vi "WLAN_be_EVM_SA_RS_CMP200.vi"(6 "SG Power":i32=-10, 7 "Function":T1, 8 "error in":errorcluster, 11 "VISA IN":refnum<visa-resource-name>="TCPIP::Vince_Wu-NB::inst0::INSTR") -> (0 "error out":errorcluster, 1 "EVM":dbl format="%#.3g", 2 "Power":dbl format="%#.3g", 3 "IDN":string)   [LabVIEW 2023, in "R_S.lvlib"]
uses:
  R_S.lvlib
  CTL/LitePoint_EVM_SA.ctl
panel:
  out "Response":string
  out "String":string
  out "EVM_ALL_Carrier_Mean":string
  out "PPDU_Power_Mean":string
  out "VSA?":string
  # "TCPIP::Vince_Wu-NB::inst0::INSTR"
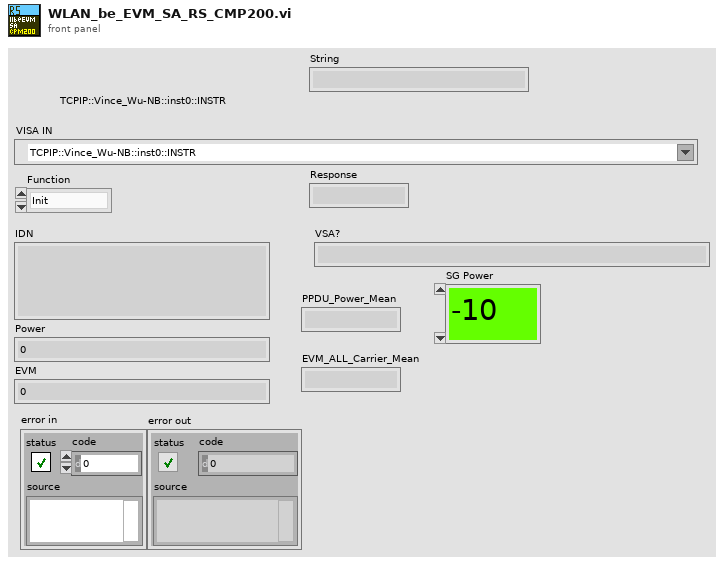
[diagram p1: front panel]
types:
  T1 = typedef "LitePoint_EVM_SA.ctl" = enum16{"Init", "Close", "set_SA", "get_EVM", "byPass", "getPower"}
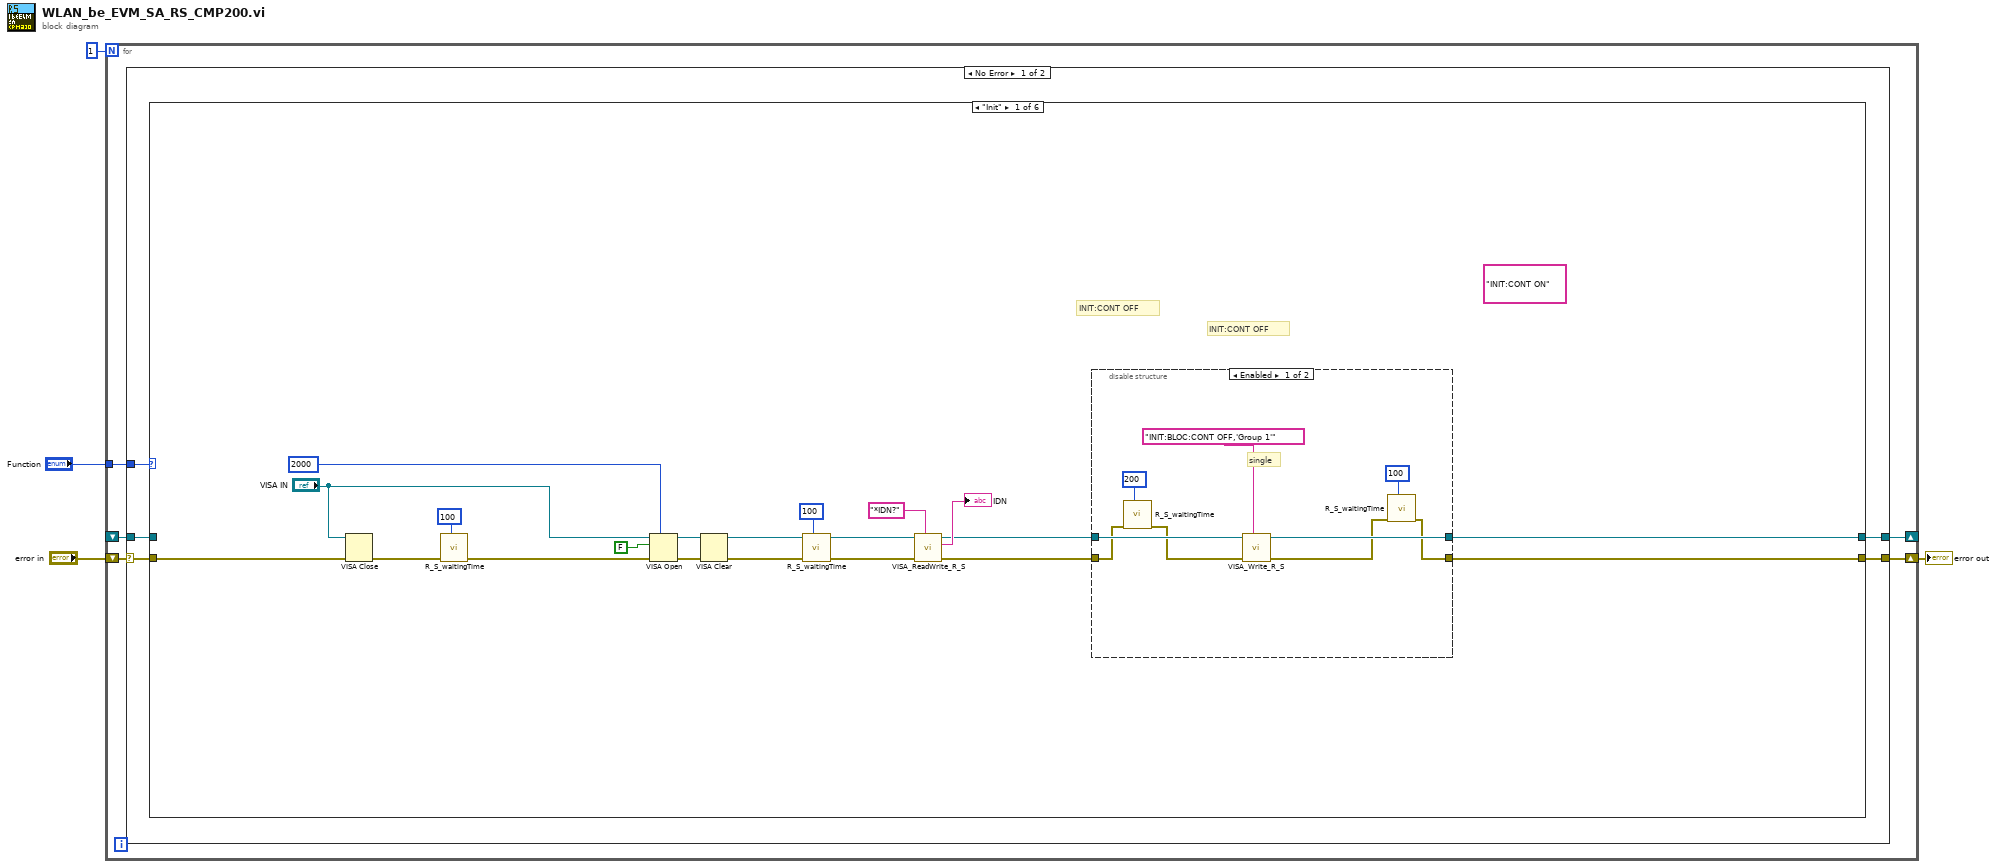
[diagram p0: block diagram]
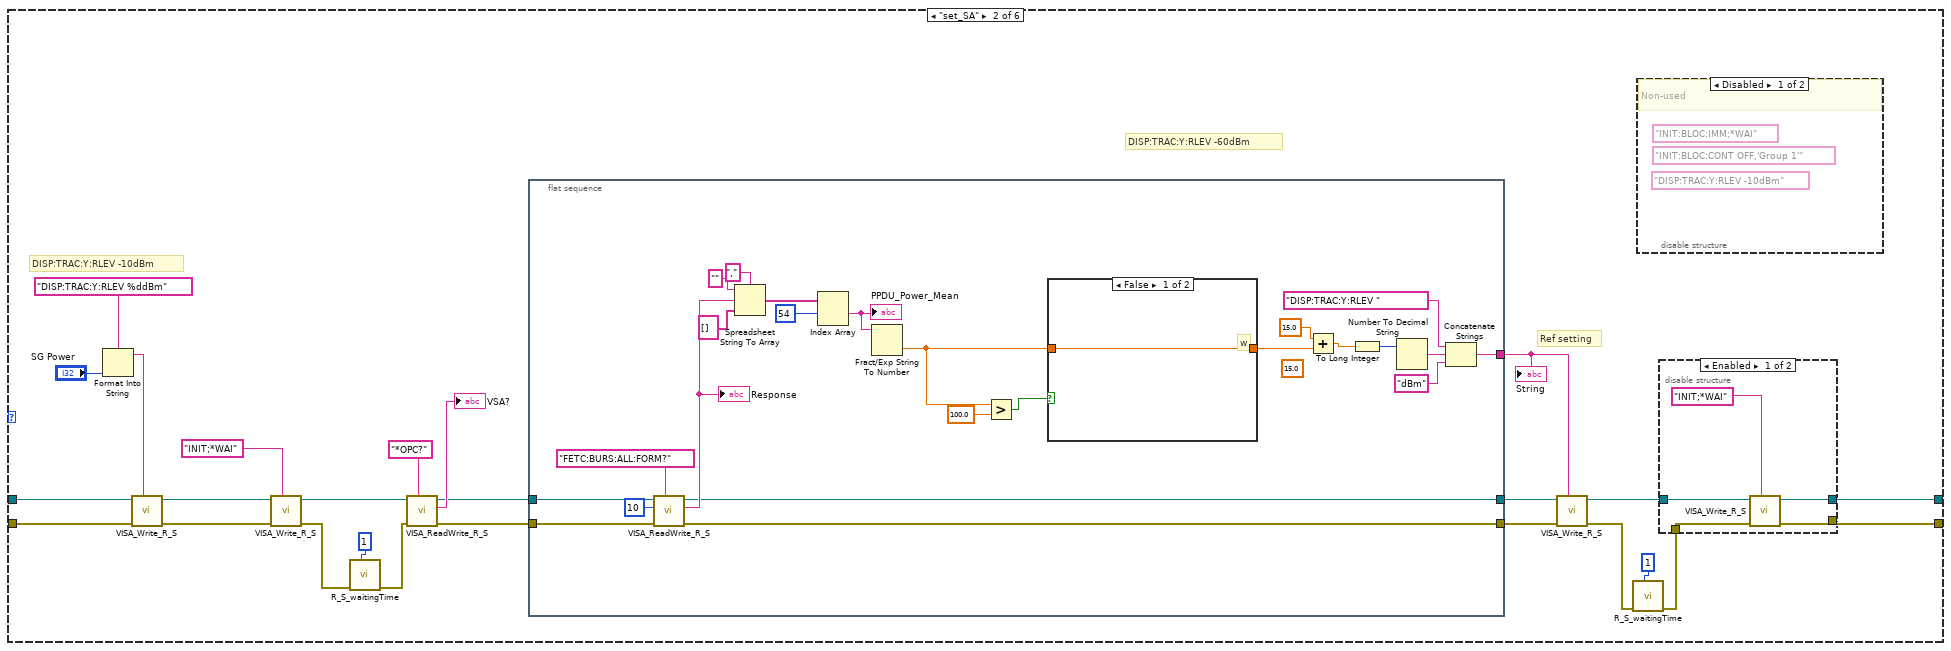
[diagram p3: hidden frame]
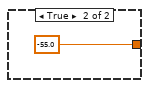
[diagram p5: hidden frame]
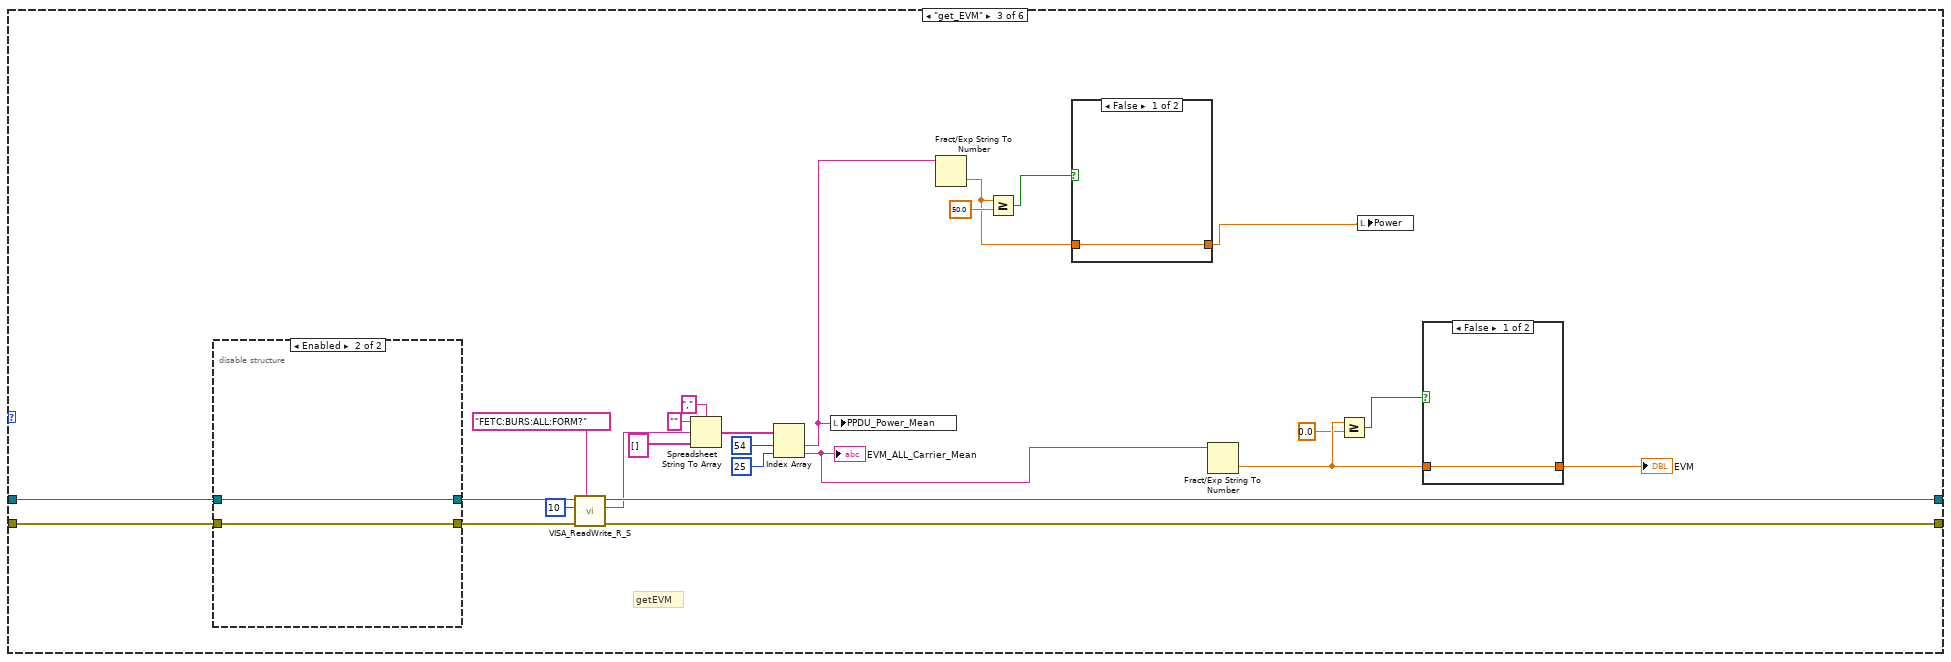
[diagram p7: hidden frame]
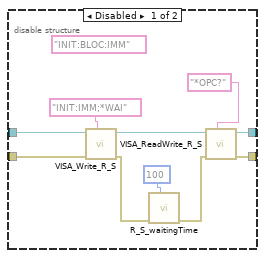
[diagram p8: hidden frame]
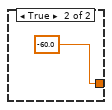
[diagram p9: hidden frame]
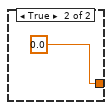
[diagram p10: hidden frame]
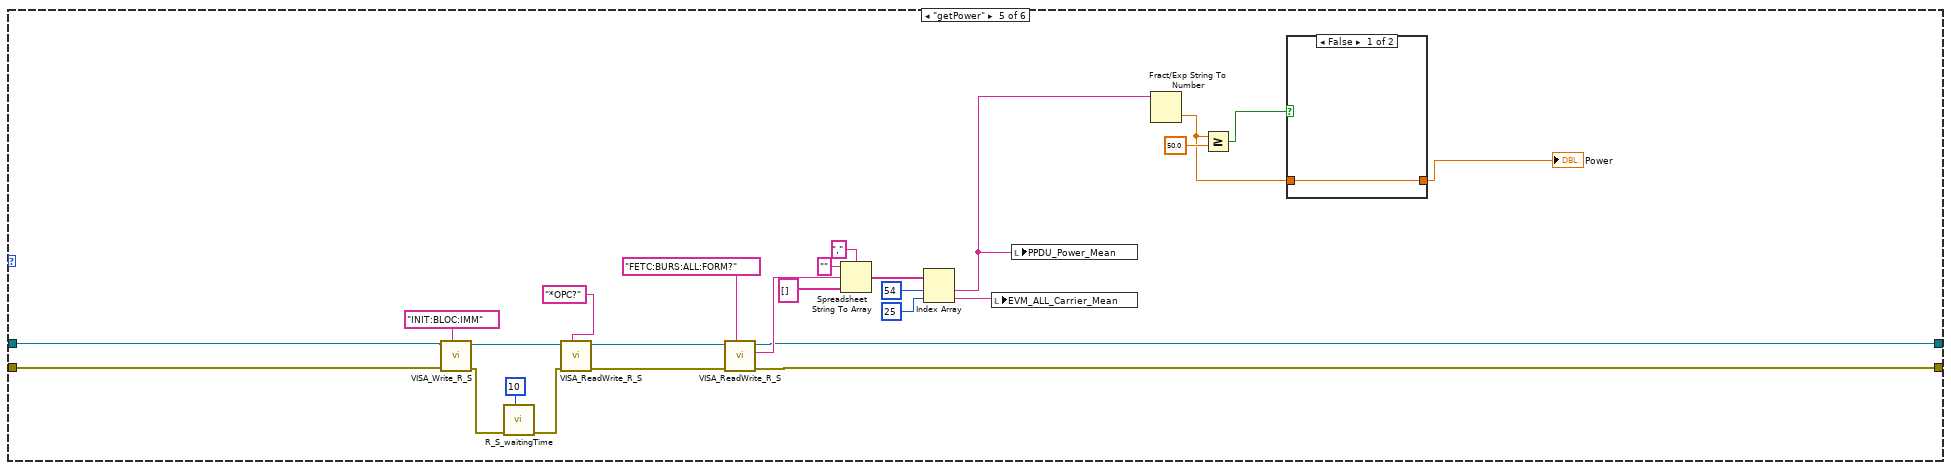
[diagram p12: hidden frame]
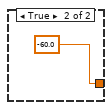
[diagram p13: hidden frame]
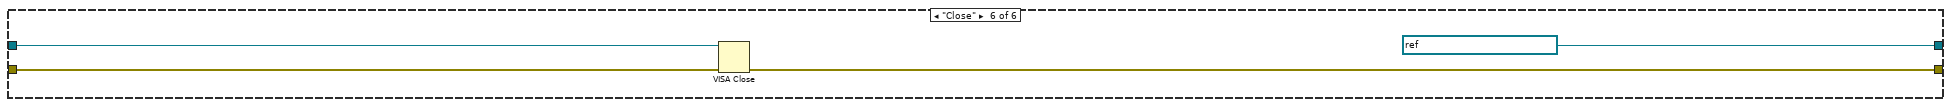
[diagram p14: hidden frame]
diagram:
  n1 = for {
    N: 1 -> [_]
    tunnel: "Function" -> [w7]
    shift-right: [w8] -> w3
    shift-left: "error in" -> [w9]
    shift-right: [w5] -> _
    shift-left: _ -> [w6]
    n2 = case shown="No Error" w9 {
      selector: w9 -> [w13 w179]
      tunnel: [w12 w179] -> w8
      tunnel: w7 -> [w14 _]
      tunnel: w6 -> [w11 w178]
      tunnel: [w10 w178] -> w5
      frame No Error {
        n3 = case shown="\"Init\"" w14 {
          tunnel: [w23 w56 w119 w145 w149 w177] -> w12
          tunnel: w13 -> [w26 w52 w120 w145 w151 w176]
          tunnel: w11 -> [_ w51 w118 w144 w152 w175]
          tunnel: [w21 w55 w117 w144 w150 refnum<visa-resource-name> refnum ("VISA out")] -> w10
          frame "Init" {
            (unwired) "INIT:CONT ON"
            # "INIT:CONT OFF"
            # "INIT:CONT OFF"
            n4 = VISA Close(VISA resource name="VISA IN", error in (no error)=w26) -> (error out=w20:errorcluster)
            n5 = call "R_S_waitingTime.vi"("Waiting Time(ms)"=u32 100, "error in"=w20) -> ("error out"=w19:errorcluster)  [unwired: 9 in]
            n6 = VISA Open(timeout (0)=u32 2000 ("VISA Open timeout (0)"), duplicate session (F)=FALSE, error in (no error)=w19, VISA resource name="VISA IN") -> (VISA resource name=w30:refnum<visa-resource-name>, error out=w31:errorcluster)  [unwired: 1 in]
            n7 = VISA Clear(VISA resource name=w30, error in (no error)=w31) -> (VISA resource name out=w29:refnum<visa-resource-name>, error out=w16:errorcluster)
            n8 = call "R_S_waitingTime.vi"("Waiting Time(ms)"=u32 100, "error in"=w16) -> ("error out"=w15:errorcluster)  [unwired: 9 in]
            n9 = call "VISA_ReadWrite_R_S.vi"("VISA_CMD"="*IDN?", "error in"=w15, "VISA in"=w29) -> ("error out"=w24:errorcluster, "Response"=→"IDN":string, "VISA out"=w22:refnum<visa-resource-name>)  [unwired: 6 in]
            n10 = disable-structure shown="Enabled" {
              disable-tunnel: w24 -> [w38 w44]
              disable-tunnel: [w35 w44] -> w23
              disable-tunnel: w22 -> [w42 w43]
              disable-tunnel: [w41 w43] -> w21
              frame Enabled {
                # "single"
                n11 = call "R_S_waitingTime.vi"("Waiting Time(ms)"=u32 200, "error in"=w38) -> ("error out"=w39:errorcluster)  [unwired: 9 in]
                n12 = call "VISA_Write_R_S.vi"("VISA CMD"="INIT:BLOC:CONT OFF,'Group 1'", "error in"=w39, "VISA in"=w42) -> ("error out"=w36:errorcluster, "VISA out"=w41:refnum<visa-resource-name>)  [unwired: 7 in]
                n13 = call "R_S_waitingTime.vi"("Waiting Time(ms)"=u32 100, "error in"=w36) -> ("error out"=w35:errorcluster)  [unwired: 9 in]
              }
              frame Disabled {
              }
            }
          }
          frame "set_SA" {
            # "DISP:TRAC:Y:RLEV -10dBm"
            # "Ref setting"
            # "DISP:TRAC:Y:RLEV -60dBm"
            n14 = Format Into String(format string="DISP:TRAC:Y:RLEV %ddBm" ("VISA CMD"), "SG Power") -> (resulting string=w45:string)  [unwired: 2 in, 1 out]
            n15 = call "VISA_Write_R_S.vi"("VISA CMD"=w45, "error in"=w52, "VISA in"=w51) -> ("error out"=w48:errorcluster, "VISA out"=w49:refnum<visa-resource-name>)  [unwired: 7 in]
            n16 = call "VISA_Write_R_S.vi"("VISA CMD"="INIT;*WAI", "error in"=w48, "VISA in"=w49) -> ("error out"=w54:errorcluster, "VISA out"=w53:refnum<visa-resource-name>)  [unwired: 7 in]
            n17 = call "R_S_waitingTime.vi"("Waiting Time(ms)"=u32 1, "error in"=w54) -> ("error out"=w69:errorcluster)  [unwired: 9 in]
            n18 = call "VISA_ReadWrite_R_S.vi"("VISA_CMD"="*OPC?", "error in"=w69, "VISA in"=w53) -> ("error out"=w65:errorcluster, "Response"=→"VSA?":string, "VISA out"=w64:refnum<visa-resource-name>)  [unwired: 6 in]
            n19 = flat-sequence {
              tunnel: w65 -> [w93]
              tunnel: w64 -> [w92]
              tunnel: [w89] -> w63
              tunnel: [w88] -> w62
              tunnel: [w87] -> w61
              frame #0 {
                (unwired) 15.0 ("x")
                n20 = call "VISA_ReadWrite_R_S.vi"("VISA_CMD"="FETC:BURS:ALL:FORM?", "error in"=w93, "waiting(ms)"=u32 10, "VISA in"=w92) -> ("error out"=w89:errorcluster, "Response"=w90:string, "VISA out"=w87:refnum<visa-resource-name>)  [unwired: 5 in]
                "Response" <- w90
                n21 = Spreadsheet String To Array(delimiter (Tab)=",", format string="", spreadsheet string=w90, array type (2D Dbl)=string[] []) -> (array=w75:string[])
                n22 = Index Array(array=w75, index #1=54 ("index")) -> (element #1=w71:string)  [unwired: 1 in, 1 out]
                "PPDU_Power_Mean" <- w71
                n23 = Fract/Exp String To Number(string=w71) -> (number=w79:dbl)  [unwired: 3 in, 1 out]
                n24 = Greater?(x=w79, y=100.0) -> (0:w77:bool)
                n25 = case shown="False" w77 {
                  tunnel: w79 -> [w94 _]
                  tunnel: [w94 -55.0 ("y")] -> w80
                  frame False {
                    # "w"
                  }
                  frame True {
                  }
                }
                n26 = Add(x=15.0, y=w80) -> (x+y=w81:dbl)
                n27 = To Long Integer(number=w81) -> (32bit integer=w70:i32)
                n28 = Number To Decimal String(number=w70) -> (decimal integer string=w83:string)  [unwired: 1 in]
                n29 = Concatenate Strings("DISP:TRAC:Y:RLEV " ("write buffer"), w83, "dBm" ("write buffer")) -> (w88:string)
              }
            }
            n30 = call "VISA_Write_R_S.vi"("VISA CMD"=w62, "error in"=w63, "VISA in"=w61) -> ("error out"=w59:errorcluster, "VISA out"=w58:refnum<visa-resource-name>)  [unwired: 7 in]
            n31 = call "R_S_waitingTime.vi"("Waiting Time(ms)"=u32 1, "error in"=w59) -> ("error out"=w57:errorcluster)  [unwired: 9 in]
            n32 = disable-structure shown="Disabled" {
              frame Disabled {
                (unwired) "DISP:TRAC:Y:RLEV -10dBm" ("VISA CMD")
                (unwired) "INIT:BLOC:IMM;*WAI"
                (unwired) "INIT:BLOC:CONT OFF,'Group 1'"
                # "Non-used"
              }
              frame Enabled {
              }
            }
            n33 = disable-structure shown="Enabled" {
              disable-tunnel: w58 -> [w100 w101]
              disable-tunnel: w57 -> [w99 w102]
              disable-tunnel: [w98 w102] -> w56
              disable-tunnel: [w97 w101] -> w55
              frame Enabled {
                n34 = call "VISA_Write_R_S.vi"("VISA CMD"="INIT;*WAI", "error in"=w99, "VISA in"=w100) -> ("error out"=w98:errorcluster, "VISA out"=w97:refnum<visa-resource-name>)  [unwired: 7 in]
              }
              frame Disabled {
              }
            }
            "String" <- w62
          }
          frame "get_EVM" {
            # "getEVM"
            n35 = disable-structure shown="Enabled" {
              disable-tunnel: [w134 w139] -> w123
              disable-tunnel: [w133 w138] -> w122
              disable-tunnel: w120 -> [w129 w139]
              disable-tunnel: w118 -> [w128 w138]
              frame Disabled {
                (unwired) "INIT:BLOC:IMM"
                n36 = call "VISA_Write_R_S.vi"("VISA CMD"="INIT:IMM;*WAI", "error in"=w129, "VISA in"=w128) -> ("error out"=w136:errorcluster, "VISA out"=w137:refnum<visa-resource-name>)  [unwired: 7 in]
                n37 = call "R_S_waitingTime.vi"("Waiting Time(ms)"=u32 100, "error in"=w136) -> ("error out"=w135:errorcluster)  [unwired: 9 in]
                n38 = call "VISA_ReadWrite_R_S.vi"("VISA_CMD"="*OPC?", "error in"=w135, "VISA in"=w137) -> ("error out"=w134:errorcluster, "VISA out"=w133:refnum<visa-resource-name>)  [unwired: 6 in, 1 out]
              }
              frame Enabled {
              }
            }
            n39 = call "VISA_ReadWrite_R_S.vi"("VISA_CMD"="FETC:BURS:ALL:FORM?", "error in"=w123, "waiting(ms)"=u32 10, "VISA in"=w122) -> ("error out"=w119:errorcluster, "Response"=w110:string, "VISA out"=w117:refnum<visa-resource-name>)  [unwired: 5 in]
            n40 = Spreadsheet String To Array(delimiter (Tab)=",", format string="", spreadsheet string=w110, array type (2D Dbl)=string[] []) -> (array=w114:string[])
            n41 = Index Array(array=w114, index #1=54 ("index"), index #2=25 ("index")) -> (element #1=w105:string, element #2=w109:string)
            "EVM_ALL_Carrier_Mean" <- w109
            n42 = local write "PPDU_Power_Mean"(w105) -> ()
            n43 = Fract/Exp String To Number(string=w105) -> (number=w106:dbl)  [unwired: 3 in, 1 out]
            n44 = Greater Or Equal?(x=w106, y=50.0) -> (x >= y?=w107:bool)
            n45 = case shown="False" w107 {
              tunnel: w106 -> [w140 _]
              tunnel: [w140 -60.0] -> w104
              frame False {
              }
              frame True {
              }
            }
            n46 = Fract/Exp String To Number(string=w109) -> (number=w126:dbl)  [unwired: 3 in, 1 out]
            n47 = Greater Or Equal?(x=w126, y=0.0) -> (x >= y?=w124:bool)
            n48 = local write "Power"(w104) -> ()
            n49 = case shown="False" w124 {
              tunnel: w126 -> [w142 _]
              tunnel: [w142 0.0] -> w127
              frame False {
              }
              frame True {
              }
            }
            "EVM" <- w127
          }
          frame "byPass", Default {
          }
          frame "getPower" {
            n50 = call "VISA_Write_R_S.vi"("VISA CMD"="INIT:BLOC:IMM", "error in"=w151, "VISA in"=w152) -> ("error out"=w166:errorcluster, "VISA out"=w167:refnum<visa-resource-name>)  [unwired: 7 in]
            n51 = call "R_S_waitingTime.vi"("Waiting Time(ms)"=u32 10, "error in"=w166) -> ("error out"=w165:errorcluster)  [unwired: 9 in]
            n52 = call "VISA_ReadWrite_R_S.vi"("VISA_CMD"="*OPC?", "error in"=w165, "VISA in"=w167) -> ("error out"=w164:errorcluster, "VISA out"=w148:refnum<visa-resource-name>)  [unwired: 6 in, 1 out]
            n53 = call "VISA_ReadWrite_R_S.vi"("VISA_CMD"="FETC:BURS:ALL:FORM?", "error in"=w164, "VISA in"=w148) -> ("error out"=w149:errorcluster, "Response"=w153:string, "VISA out"=w150:refnum<visa-resource-name>)  [unwired: 6 in]
            n54 = Spreadsheet String To Array(delimiter (Tab)=",", format string="", spreadsheet string=w153, array type (2D Dbl)=string[] []) -> (array=w157:string[])
            n55 = Index Array(array=w157, index #1=54 ("index"), index #2=25 ("index")) -> (element #1=w146:string, element #2=w147:string)
            n56 = local write "EVM_ALL_Carrier_Mean"(w147) -> ()
            n57 = local write "PPDU_Power_Mean"(w146) -> ()
            n58 = Fract/Exp String To Number(string=w146) -> (number=w169:dbl)  [unwired: 3 in, 1 out]
            n59 = Greater Or Equal?(x=w169, y=50.0) -> (x >= y?=w170:bool)
            n60 = case shown="False" w170 {
              tunnel: w169 -> [w172 _]
              tunnel: [w172 -60.0] -> w168
              frame False {
              }
              frame True {
              }
            }
            "Power" <- w168
          }
          frame "Close" {
            n61 = VISA Close(VISA resource name=w175, error in (no error)=w176) -> (error out=w177:errorcluster)
          }
        }
      }
      frame Error {
      }
    }
  }
  "error out" <- w3
